vi "PicoScope2000aGetValues.vi"(5 "Segment Range":T1 {"toSegmentIndex" format="%.4p"; "fromSegmentIndex" format="%.4p"}, 7 "Buffer and Transfer Settings":T2={"startIndex"=0, "Samples"=1000, "Down Sample Ratio"=1, "Down-Sample Mode"=1} {"Down-Sample Mode" items=["RAW none"=2147483648, "None"=0, "Aggregate"=1, "Decimate"=2, "Average"=4]; "Down Sample Ratio" step=1; "Samples" format="%_6p"}, 8 "error in (no error)":errorcluster, 11 "handle in":i16) -> (0 "error out":errorcluster, 3 "handle out":i16, 4 "overflow":i16 format="%010b", 6 "noOfSamples":u64)   [LabVIEW 2010]
doc: "Calls ps2000aGetValues"
uses:
  ps2000a.dll
  shared/Buffer and Transfer Settings.ctl
  shared/Segment Range.ctl
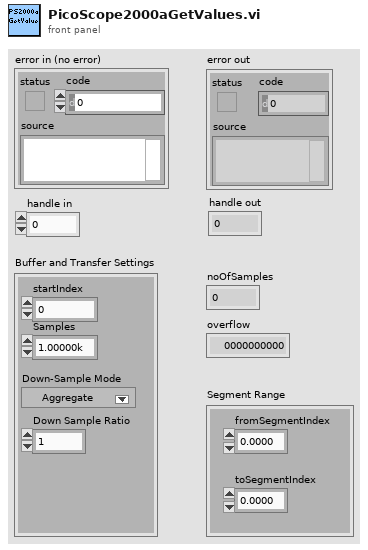
[diagram p1: front panel]
types:
  T1 = typedef "Segment Range.ctl" = cluster{"fromSegmentIndex":u64, "toSegmentIndex":u64}
  T2 = typedef "Buffer and Transfer Settings.ctl" = cluster{"startIndex":u64, "Samples":u64, "Down Sample Ratio":u64, "Down-Sample Mode":u32}
  T3 = cluster{"status":bool, "code":u32, "source":string}
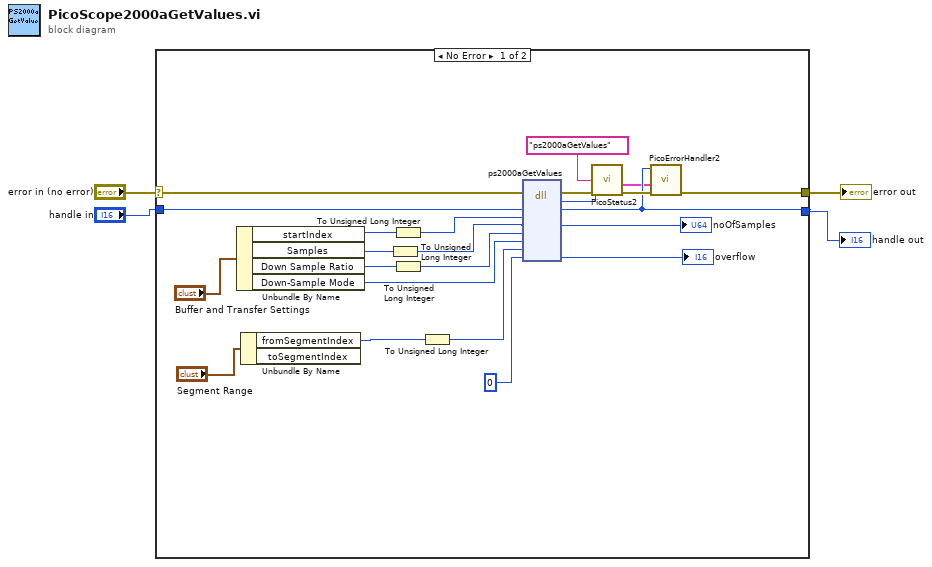
[diagram p0: block diagram]
diagram:
  n1 = case shown="No Error" "error in (no error)" {
    selector: "error in (no error)" -> [w22 w28]
    tunnel: "handle in" -> [w21 w29]
    tunnel: [w6 w29] -> w4
    tunnel: [w20 w28] -> w3
    frame No Error {
      n2 = Unbundle By Name("Buffer and Transfer Settings") -> ("startIndex"=w14:u64, "Samples"=w12:u64, "Down Sample Ratio"=w13:u64, "Down-Sample Mode"=w8:u32)
      n3 = Unbundle By Name("Segment Range") -> ("fromSegmentIndex"=w16:u64)  [unwired: 1 out]
      n4 = To Unsigned Long Integer(number=w12) -> (unsigned 32bit integer=w10:u32)
      n5 = To Unsigned Long Integer(number=w14) -> (unsigned 32bit integer=w11:u32)
      n6 = To Unsigned Long Integer(number=w13) -> (unsigned 32bit integer=w9:u32)
      n7 = To Unsigned Long Integer(number=w16) -> (unsigned 32bit integer=w15:u32)
      n8 = dll-call lib="ps2000a.dll" fn="ps2000aGetValues" ("ps3000.dll:_ps3000_open_unit@0")(error in=w22, "handle"=w21, "startIndex"=w11, "noOfSamples"=w10, "downSampleRatio"=w9, "downSampleRatioMode"=w8, "segmentIndex"=w15, "overflow"=i16 0) -> (error out=w26:errorcluster, "PICO_STATUS"=w7:u32, "handle"=w6:i16, "noOfSamples"=→"noOfSamples":u32, "overflow"=→"overflow":i16)  [unwired: 6 in, 1 out]
      n9 = call "PicoStatus2.vi"("PICO source"="ps2000aGetValues" ("source"), "Error in"=w26, "PICO STATUS"=w7) -> ("error out"=w27:errorcluster, "PICO_STATUS out"=w5:T3)  [unwired: 5 in]
      n10 = call "PicoErrorHandler2.vi"("error in (no error)"=w27, "PICO_STATUS in"=w5, "handle In"=w6) -> ("error out"=w20:errorcluster)  [unwired: 8 in]
    }
    frame Error {
    }
  }
  "error out" <- w3
  "handle out" <- w4
